vi "Open Flags to Flags.vi"(1 "open flags":T1) -> (0 "flags":u32 format="%08x")   [LabVIEW 2020, in "NI_SFTP.lvlib" / "SSH_FXP_OPEN.lvclass"]
uses:
  <vilib>/net/SFTP/API/Support/Command/SSH_FXP_OPEN/SSH_FXP_OPEN.lvclass
  <vilib>/net/SFTP/API/Support/Open Flags.ctl
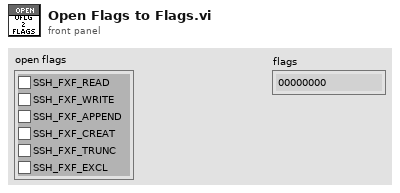
[diagram p1: front panel]
types:
  T1 = typedef "NI_SFTP.lvlib/SSH_FXP_OPEN.lvclass/Open Flags.ctl" = cluster{"SSH_FXF_READ":bool, "SSH_FXF_WRITE":bool, "SSH_FXF_APPEND":bool, "SSH_FXF_CREAT":bool, "SSH_FXF_TRUNC":bool, "SSH_FXF_EXCL":bool}
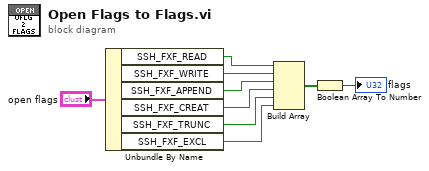
[diagram p0: block diagram]
diagram:
  n1 = Unbundle By Name("open flags") -> ("SSH_FXF_READ"=w7:bool, "SSH_FXF_WRITE"=w6:bool, "SSH_FXF_APPEND"=w5:bool, "SSH_FXF_CREAT"=w4:bool, "SSH_FXF_TRUNC"=w3:bool, "SSH_FXF_EXCL"=w2:bool)
  n2 = Build Array(w7, w6, w5, w4, w3, w2) -> (w1:bool[])
  n3 = Boolean Array To Number(Boolean array=w1) -> (number=→"flags":u8)
